vi "Bypass Measure Layer Control.vi"(8 "error in (no error)":errorcluster, 10 "Measure Bypass Option (0: Immediate)":i32(ring) items=["Immediate", "Signal"], 11 "VISA resource name":refnum<visa-resource-name>) -> (0 "error out":errorcluster, 3 "VISA resource name out":refnum<visa-resource-name>)   [LabVIEW 2016, in "Keithley 6517.lvlib"]
doc: "Bypasses the arm, scan, and measure control source and delays for the Measure Layer (Trigger) of the trigger model. You can use it when you do not wish to wait for the programmed event.\n\nNote:\nThe instrument must be waiting for the appropriate event when this command is sent. Otherwise, an error occurs and the command is ignored. When the command is sent, the bypass occurs and operation continues on.\n\nThis VI is <B>NOT</B> compatible with model <B>6514</B>."
uses:
  <instrlib>/Keithley 6517/Keithley 6517.lvlib
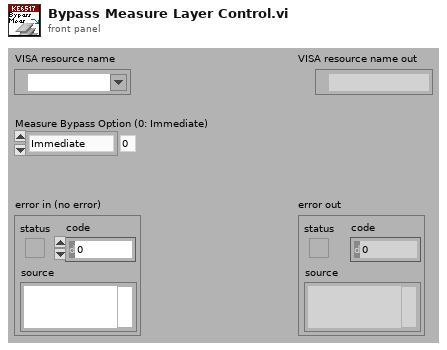
[diagram p1: front panel]
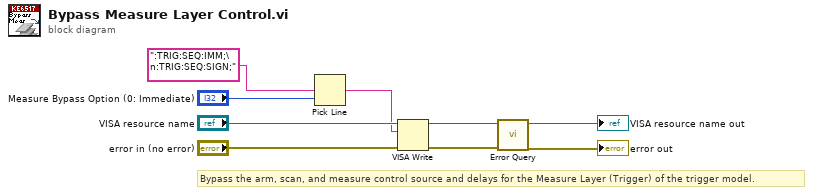
[diagram p0: block diagram]
diagram:
  # "Bypass the arm, scan, and measure control source and delays for the Measure Layer (Trigger) of the trigger model."
  n1 = Pick Line(multi-line string=":TRIG:SEQ:IMM;\n:TRIG:SEQ:SIGN;", line index="Measure Bypass Option (0: Immediate)") -> (output string=w1:string)  [unwired: 1 in]
  n2 = VISA Write(VISA resource name="VISA resource name", write buffer=w1, error in (no error)="error in (no error)") -> (VISA resource name out=w7:refnum<visa-resource-name>, error out=w6:errorcluster)  [unwired: 1 out]
  n3 = call <instrlib>:"Error Query.vi"("error in (no error)"=w6, "VISA resource name"=w7) -> ("error out"=→"error out":errorcluster, "VISA resource name out"=→"VISA resource name out":refnum<visa-resource-name>)  [unwired: 6 in, 2 out]
